vi "Build Broadcast Msg.vi"(8 "error in (no error)":errorcluster, 10 "Brower Controller_Q":refnum<class "Message Enqueuer.lvclass">, 11 "Button Builder.lvclass":refnum<class "Button_Builder.lvclass">) -> (0 "error out":errorcluster, 3 "Button Builder.lvclass out":refnum<class "Button_Builder.lvclass">)   [LabVIEW 2015, in "Button_Builder.lvclass"]
uses:
  Button_Builder.lvclass
  <vilib>/ActorFramework/Message Enqueuer/Message Enqueuer.lvclass
  GUI Control Builder/GUI Control Builder.lvclass/GUI Control Builder.ctl
  GUI Controls/GUI Control/GUI Control.lvclass/GUI Control.ctl
  Browers/Browers Controller Messages/Add Contents In Tree Msg/Add Contents In Tree Msg.lvclass/Add Contents In Tree Msg.ctl
  <vilib>/ActorFramework/Message Enqueuer/Message Enqueuer.lvclass/Message Enqueuer.ctl
  <vilib>/ActorFramework/Message Enqueuer/Enqueue.vi
  <vilib>/ActorFramework/Message Priority Queue/Priority Enqueue.vi
  GUI Controls/GUI Control/GUI Control.lvclass
  Browers/Browers Controller Messages/Add Contents In Tree Msg/Add Contents In Tree Msg.lvclass
  GUI Control Builder/GUI Control Builder.lvclass
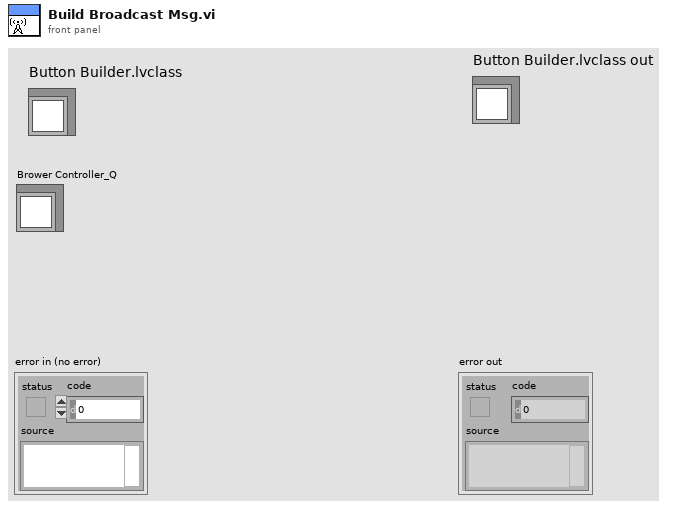
[diagram p1: front panel]
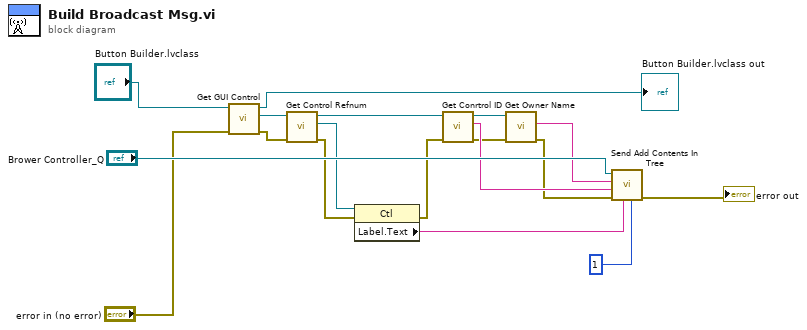
[diagram p0: block diagram]
diagram:
  n1 = call "Get GUI Control.vi"("error in (no error)"="error in (no error)", "Control Builder in"="Button Builder.lvclass") -> ("error out"=w9:errorcluster, "GUI Control"=w16:refnum<class "GUI Control.lvclass">, "Control Builder out"=→"Button Builder.lvclass out":refnum<class "Button_Builder.lvclass">)  [unwired: 7 in]
  n2 = call "Get Control Refnum.vi"("error in (no error)"=w9, "GUI Control in"=w16) -> ("error out"=w8:errorcluster, "Ctl Refnum"=w14:refnum<vi>, "GUI Control out"=w15:refnum<class "GUI Control.lvclass">)  [unwired: 7 in]
  n3 = property class="Ctl"(reference=w14, error in=w8) -> (error out=w7:errorcluster, "Label.Text"=w11:string)  [unwired: 1 out]
  n4 = call "Get Conrtrol ID.vi"("error in (no error)"=w7, "GUI Control in"=w15) -> ("error out"=w6:errorcluster, "Control ID"=w10:string, "GUI Control out"=w13:refnum<class "GUI Control.lvclass">)  [unwired: 7 in]
  n5 = call "Get Owner Name.vi"("error in (no error)"=w6, "GUI Control in"=w13) -> ("error out"=w5:errorcluster, "Owner Name"=w12:string)  [unwired: 7 in, 1 out]
  n6 = call "Send Add Contents In Tree.vi"("Symbol Index"=1, "Node Name"=w11, "error in (no error)"=w5, "Node ID"=w10, "Parent Node"=w12, "Message Enqueuer"="Brower Controller_Q") -> ("error out"=→"error out":errorcluster)  [unwired: 4 in, 1 out]
